vi "BB_CameraOpen.vi"(8 "error in (no error)":errorcluster, 11 "Camera Address":string="192.168.0.90") -> (0 "error out":errorcluster, 3 "CameraDevRef":T1)   [LabVIEW 2015]
doc: "Opens a reference to the camera you specify. This reference can then be used with the other functions on the camera palette. If a reference to the camera is already open, this VI returns an error.\n\nThis software is licensed. Open the labview\\readme\\WPI Robotics Library Open Source License.txt file for more information."
uses:
  <vilib>/Rock Robotics/WPI/Camera/WPI_CameraDevRef.ctl
  <vilib>/Rock Robotics/WPI/Camera/WPI_CameraRegistryActions.ctl
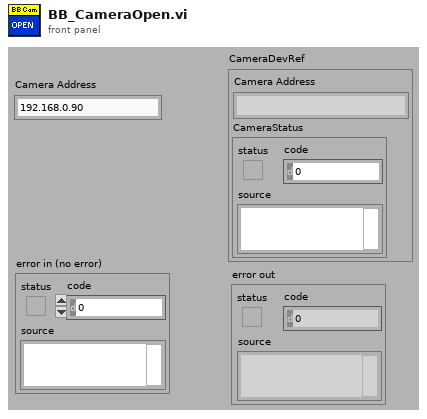
[diagram p1: front panel]
types:
  T1 = typedef "WPI_CameraDevRef.ctl" = cluster{"Camera Address":string, "CameraStatus":errorcluster}
  T2 = typedef "WPI_CameraRegistryActions.ctl" = enum16{"Open", "Close"}
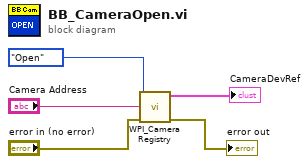
[diagram p0: block diagram]
diagram:
  n1 = call <vilib>:"WPI_Camera Registry.vi"("error in (no error)"="error in (no error)", "Camera Address"="Camera Address", "Action"=WPI_CameraRegistryActions."Open" ("Enum")) -> ("error out"=→"error out":errorcluster, "CameraDevRef"=→"CameraDevRef":T1)  [unwired: 1 in, 6 out]
